vi "Networktable comms.vi"   [LabVIEW 2013]
uses:
  Events.vi
panel:
  # "This is for All network table communications"
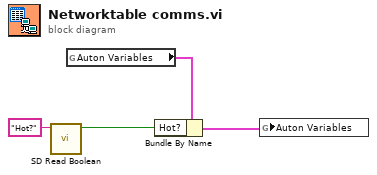
[diagram p0: block diagram]
diagram:
  n1 = call <vilib>:"SD Read Boolean.vi"("Name"="Hot?") -> ("Boolean"=w2:bool)  [unwired: 8 in, 2 out]
  n2 = global read "Events.vi" "Auton Variables"() -> (w3:cluster{"Hot?":bool})
  n3 = Bundle By Name(cluster=w3, "Hot?"=w2) -> (w4:cluster{"Hot?":bool})
  n4 = global write "Events.vi" "Auton Variables"(w4) -> ()
